vi "MAIN.vi"() -> ()   [LabVIEW 2024]
panel:
  out "error out":errorcluster
  in  "Error In":errorcluster
  in  "Tab Control":enum32{"MAIN"}(tab)
  in  "Tab Control 2":enum32{"LOGIN"}(tab)
  in  "Copy Button":bool
  in  "OK Button":bool
  in  "PASSWORD":string
  in  "USER ID":string
  in  "Jump Button":bool
  in  "Stop Button":bool
  in  "Play Button":bool
  in  "Settings Button":bool
  in  "First Button":bool
  in  "Last Button":bool
  out "DB":bool
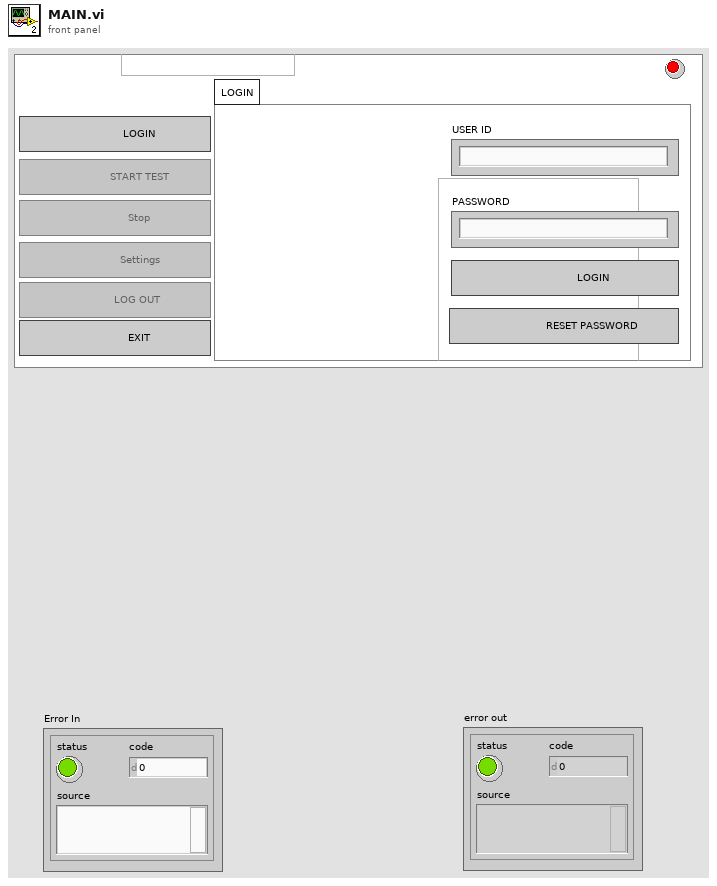
[diagram p1: front panel]
types:
  T1 = enum8{"Enabled", "Disabled", "Disabled and Grayed Out"}
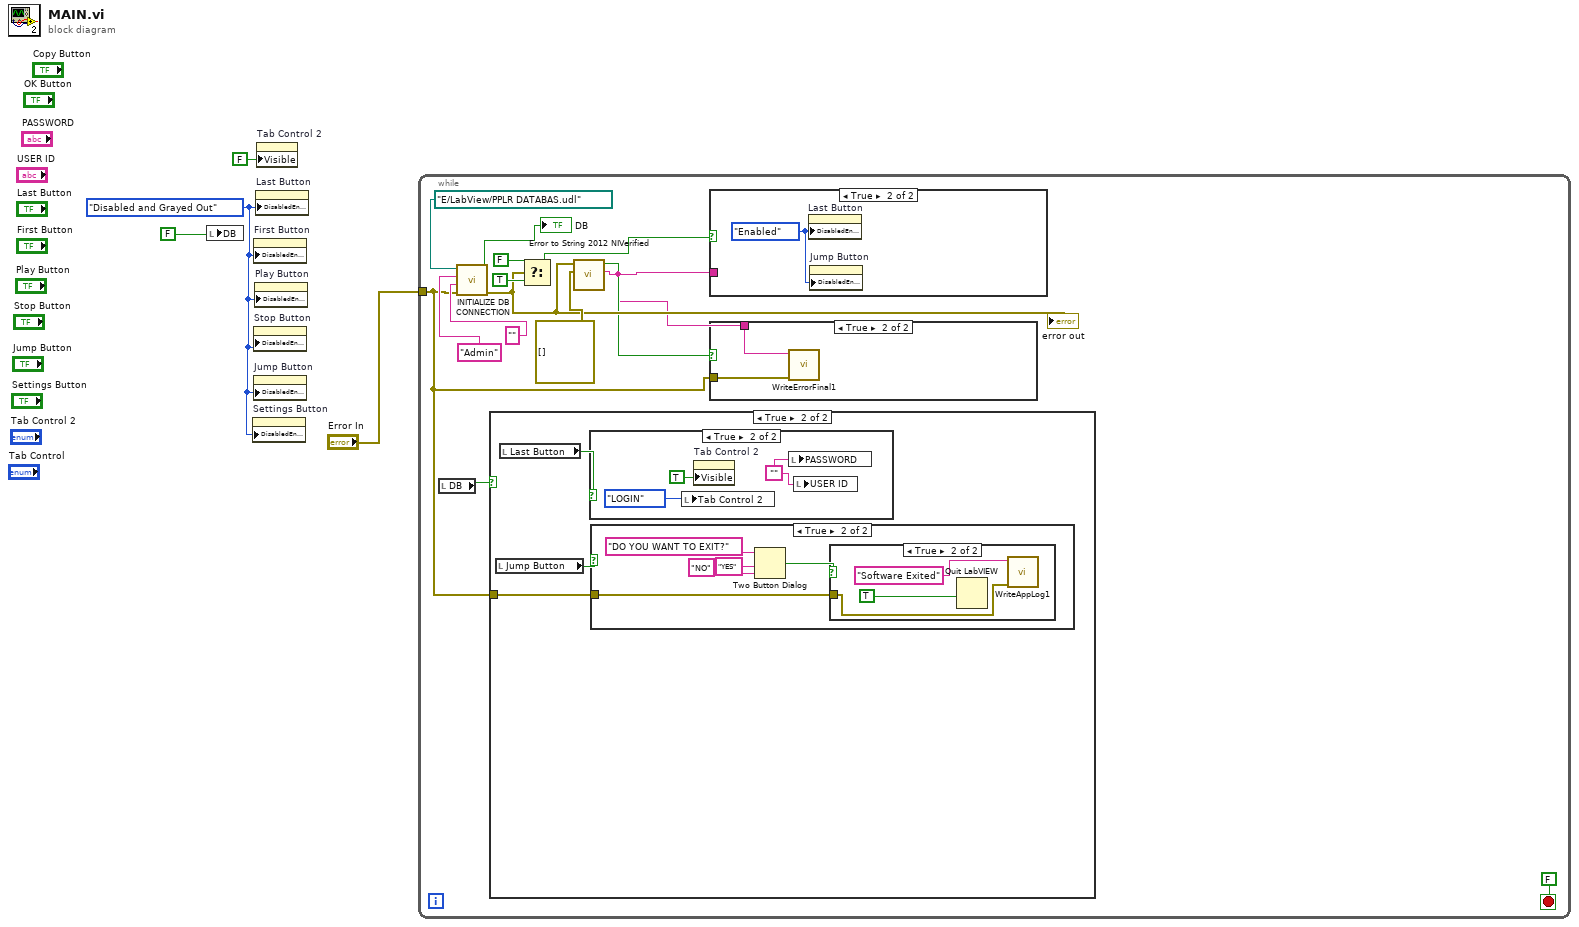
[diagram p0: block diagram]
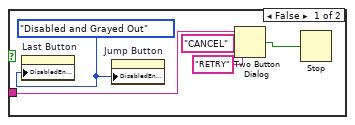
[diagram p7: hidden frame]
diagram:
  w3 = T1."Disabled and Grayed Out" ("Disabled")
  n1 = local write "DB"(FALSE) -> ()
  n2 = property on="Settings Button" class="Bool"("DisabledEnum"=w3) -> ()  [unwired: 2 in, 2 out]
  n3 = property on="First Button" class="Bool"("DisabledEnum"=w3) -> ()  [unwired: 2 in, 2 out]
  n4 = property on="Stop Button" class="Bool"("DisabledEnum"=w3) -> ()  [unwired: 2 in, 2 out]
  n5 = property on="Jump Button" class="Bool (strict)"("DisabledEnum"=w3) -> ()  [unwired: 2 in, 2 out]
  n6 = property on="Play Button" class="Bool"("DisabledEnum"=w3) -> ()  [unwired: 2 in, 2 out]
  n7 = property on="Last Button" class="Bool (strict)"("DisabledEnum"=w3) -> ()  [unwired: 2 in, 2 out]
  n8 = property on="Tab Control 2" class="TabCtl (strict)"("Visible"=FALSE) -> ()  [unwired: 2 in, 2 out]
  n9 = while {
    tunnel: "Error In" -> [w5]
    stop <- FALSE stop-if-true
    n10 = local read "DB"() -> (w7:bool)
    n11 = call "INITIALIZE DB CONNECTION.vi"("error in (no error)"=w5, "Password"="", "User Name"="Admin", "DB PATH"=path "E:/LabView/PPLR DATABAS.udl") -> ("error out"=w10:errorcluster, "CONNECTED?"=→"DB":bool)  [unwired: 6 in]
    "error out" <- w10
    n12 = case shown="True" w7 {
      tunnel: w5 -> [_ w19]
      frame False {
      }
      frame True {
        n13 = local read "Jump Button"() -> (w20:bool)
        n14 = local read "Last Button"() -> (w21:bool)
        n15 = case shown="True" w21 {
          frame False {
          }
          frame True {
            w30 = ""
            n16 = local write "Tab Control 2"(enum32{"LOGIN", "Page 2"}."LOGIN" ("Tab Control 2")) -> ()
            n17 = property on="Tab Control 2" class="TabCtl (strict)"("Visible"=TRUE) -> ()  [unwired: 2 in, 2 out]
            n18 = local write "PASSWORD"(w30) -> ()
            n19 = local write "USER ID"(w30) -> ()
          }
        }
        n20 = case shown="True" w20 {
          tunnel: w19 -> [_ w22]
          frame False {
          }
          frame True {
            n21 = Two Button Dialog(message="DO YOU WANT TO EXIT?", 1:"NO" ("F button name (\"Cancel\")"), 2:"YES" ("T button name (\"OK\")")) -> (T button?=w23:bool)
            n22 = case shown="True" w23 {
              tunnel: w22 -> [_ w27]
              frame False {
              }
              frame True {
                n23 = Quit LabVIEW(quit? (T)=TRUE) -> ()
                n24 = call "WriteAppLog1.vi"("error in (no error)"=w27, "Msg"="Software Exited") -> ()  [unwired: 9 in, 1 out]
              }
            }
          }
        }
      }
    }
    n25 = Select(t=FALSE, s=w10, f=TRUE) -> (s? t:f=w13:bool)
    n26 = call "Error to String 2012 NIVerified.vi"("Error Array"=errorcluster[] [], "Error In"=w10) -> ("Errors Strings"=w8:string, "Errors status"=w9:bool)  [unwired: 8 in]
    n27 = case shown="True" w13 {
      tunnel: w8 -> [w38 _]
      frame False {
        w39 = T1."Disabled and Grayed Out" ("Disabled")
        n28 = property on="Last Button" class="Bool (strict)"("DisabledEnum"=w39) -> ()  [unwired: 2 in, 2 out]
        n29 = property on="Jump Button" class="Bool (strict)"("DisabledEnum"=w39) -> ()  [unwired: 2 in, 2 out]
        n30 = Two Button Dialog(message=w38, 1:"RETRY" ("F button name (\"Cancel\")"), 2:"CANCEL") -> (T button?=w35:bool)
        n31 = Stop(stop? (T)=w35) -> ()
      }
      frame True {
        w40 = T1."Enabled" ("Disabled")
        n32 = property on="Last Button" class="Bool (strict)"("DisabledEnum"=w40) -> ()  [unwired: 2 in, 2 out]
        n33 = property on="Jump Button" class="Bool (strict)"("DisabledEnum"=w40) -> ()  [unwired: 2 in, 2 out]
      }
    }
    n34 = case shown="True" w9 {
      tunnel: w8 -> [_ w34]
      tunnel: w5 -> [_ w33]
      frame False {
      }
      frame True {
        n35 = call "WriteErrorFinal1.vi"("error in (no error)"=w33, "Error"=w34) -> ()  [unwired: 9 in, 1 out]
      }
    }
  }
